vi "Lab Panel V5.11.vi"() -> ()   [LabVIEW 2013] (continued)
                      tunnel: w5311 -> [w5327 _]
                      tunnel: [w5326 FALSE] -> w5294
                      frame False {
                        n2899 = Equal?(x=w5328, y=w5327) -> (x = y?=w5326:bool)
                      }
                      frame True {
                      }
                    }
                    n2900 = Or(x=w5295, y=w5294) -> (x .or. y?=w5289:bool)
                    n2901 = Or(x=w5293, y=w5292) -> (x .or. y?=w5288:bool)
                    n2902 = Or(x=w5296, y=w5297) -> (x .or. y?=w5284:bool)
                    n2903 = Or(x=w5289, y=w5288) -> (x .or. y?=w5287:bool)
                    n2904 = Or(x=w5286, y=w5287) -> (x .or. y?=w5285:bool)
                    n2905 = Or(x=w5285, y=w5284) -> (x .or. y?=w5283:bool)
                  }
                  frame #3 {
                    n2906 = local read "on loops"() -> (w5366:dbl)
                    n2907 = local read "jig cycle"() -> (w5363:dbl)
                    n2908 = local read "Send Mail Now"() -> (w5357:bool)
                    n2909 = Add(x=w5366, y=3.0) -> (x+y=w5364:dbl)
                    n2910 = Equal?(x=w5363, y=w5364) -> (x = y?=w5358:bool)
                    n2911 = And(x=w5358, y=w5357) -> (x .and. y?=w5356:bool)
                    n2912 = And(x=w5362, y=w5358) -> (x .and. y?=w5361:bool)
                    n2913 = And(x=w5361, y=w5360) -> (x .and. y?=w5359:bool)
                    n2914 = Or(x=w5359, y=w5356) -> (x .or. y?=w5355:bool)
                    n2915 = case shown="True" w5355 {
                      tunnel: w5371 -> [_ w5377]
                      tunnel: w5370 -> [_ w5376]
                      tunnel: "Lab Panel Test Status" -> [_ w5375]
                      tunnel: w5368 -> [_ w5374]
                      tunnel: w5367 -> [_ w5373]
                      tunnel: w5354 -> [_ w5372]
                      frame False {
                      }
                      frame True {
                        n2916 = stacked-sequence {
                          tunnel: w5377 -> [w5385 _]
                          tunnel: w5376 -> [w5384 _]
                          tunnel: w5375 -> [w5383 _]
                          tunnel: w5374 -> [w5382 _]
                          tunnel: w5373 -> [w5381 _]
                          tunnel: w5372 -> [w5380 _]
                          frame #0 {
                            n2917 = call "sub vi - send mail v5.vi"("TO:"=w5385, "subject"=w5383, "from"=w5381, "out going server"=w5382, "message"=w5384) -> ("error out"=w5379:errorcluster)  [unwired: 10 in]
                            n2918 = Bundle(cluster=w5380, "mail error"=w5379) -> (w5378:T7)  [unwired: 6 in]
                            n2919 = local write "MAIL SETTINGS"(w5378) -> ()
                          }
                          frame #1 {
                            n2920 = local write "mail control"("") -> ()
                            n2921 = local write "Send Mail Now"(FALSE) -> ()
                          }
                        }
                      }
                    }
                  }
                }
              }
            }
          }
          frame #18 {
            # "save jig cycle values once all run switches are off"
            n2922 = stacked-sequence {
              tunnel: w5397 -> [_ w5426]
              tunnel: w5396 -> [_ w5425]
              tunnel: w5395 -> [_ w5424]
              tunnel: w5394 -> [_ w5423]
              tunnel: w5393 -> [_ w5422]
              tunnel: w5392 -> [_ w5421]
              tunnel: w5391 -> [_ w5420]
              tunnel: w5390 -> [_ w5419]
              tunnel: w5389 -> [_ w5418]
              tunnel: w5388 -> [_ w5417]
              frame #0 {
              }
              frame #1 {
                n2923 = Not(x=w5417) -> (.not. x?=w5400:bool)
                n2924 = Not(x=w5425) -> (.not. x?=w5415:bool)
                n2925 = Not(x=w5422) -> (.not. x?=w5410:bool)
                n2926 = Not(x=w5420) -> (.not. x?=w5406:bool)
                n2927 = Not(x=w5418) -> (.not. x?=w5402:bool)
                n2928 = Not(x=w5426) -> (.not. x?=w5416:bool)
                n2929 = Not(x=w5424) -> (.not. x?=w5414:bool)
                n2930 = Not(x=w5421) -> (.not. x?=w5408:bool)
                n2931 = Not(x=w5423) -> (.not. x?=w5412:bool)
                n2932 = Not(x=w5419) -> (.not. x?=w5404:bool)
                n2933 = local read "Save JC"() -> (w5428:bool)
                n2934 = And(x=w5416, y=w5415) -> (x .and. y?=w5413:bool)
                n2935 = And(x=w5413, y=w5414) -> (x .and. y?=w5411:bool)
                n2936 = And(x=w5411, y=w5412) -> (x .and. y?=w5409:bool)
                n2937 = And(x=w5409, y=w5410) -> (x .and. y?=w5407:bool)
                n2938 = And(x=w5407, y=w5408) -> (x .and. y?=w5405:bool)
                n2939 = And(x=w5405, y=w5406) -> (x .and. y?=w5403:bool)
                n2940 = And(x=w5403, y=w5404) -> (x .and. y?=w5401:bool)
                n2941 = And(x=w5401, y=w5402) -> (x .and. y?=w5399:bool)
                n2942 = And(x=w5399, y=w5400) -> (x .and. y?=w5398:bool)
                n2943 = And(x=w5398, y=w5428) -> (x .and. y?=w5427:bool)
                n2944 = case shown="True" w5427 {
                  tunnel: w5398 -> [w5429 _]
                  frame False {
                    n2945 = case shown="False" w5429 {
                      frame False {
                        n2946 = local write "Save JC"(TRUE) -> ()
                      }
                      frame True {
                      }
                    }
                  }
                  frame True {
                    n2947 = stacked-sequence {
                      frame #0 {
                        n2948 = String To Path(string="c:\\crabtree\\Jig Cycles\\") -> (path=w5441:path)
                        n2949 = Build Path(base path=w5441, name or relative path="jigcycles.bin") -> (appended path=w5439:path)
                        n2950 = Create Folder(path (use dialog)=w5441) -> (error out=w5443:errorcluster)  [unwired: 2 in, 2 out]
                        n2951 = local read "JIG RELAY CYCLES"() -> (w5433:T8)
                        n2952 = call <vilib>:"Clear Errors.vi"("error in (no error)"=w5443) -> ()  [unwired: 6 in, 1 out]
                        n2953 = local write "Save JC"(FALSE) -> ()
                        n2954 = Open/Create/Replace File(file path (use dialog)=w5439, operation (0:open)=T21."replace or create") -> (refnum out=w5437:refnum<file>, error out=w5438:errorcluster)  [unwired: 4 in, 1 out]
                        n2955 = Write to Binary File(file (use dialog)=w5437, data=w5433, error in=w5438) -> (refnum out=w5436:refnum<file>, error out=w5435:errorcluster)  [unwired: 3 in, 1 out]
                        n2956 = Close File(refnum=w5436, error in=w5435) -> (error out=w5434:errorcluster)  [unwired: 1 out]
                        n2957 = local write "data file error"(w5434) -> ()
                      }
                      frame #1 {
                        n2958 = local read "JIG RELAY CYCLES"() -> (w5466:T8)
                        n2959 = Unbundle By Name(w5466) -> ("LAB01-1"=w5461:dbl, "LAB01-2"=w5460:dbl, "LAB02-1"=w5458:dbl, "LAB02-2"=w5457:dbl, "LAB03-1"=w5455:dbl, "LAB03-2"=w5452:dbl, "LAB04-1"=w5451:dbl, "LAB04-2"=w5449:dbl, "LAB05-1"=w5447:dbl, "LAB05-2"=w5445:dbl)
                        n2960 = stacked-sequence {
                          tunnel: w5461 -> [w5469 _ _ _ _ _ _ _ _ _]
                          tunnel: 1000000 -> [w5472 w5482 w5492 w5502 w5512 w5522 w5532 w5542 w5552 w5562]
                          tunnel: [w5470 _ _ _ _ _ _ _ _ _] -> w5464
                          tunnel: "TEST STATION HAS REACHED 1 MILLION CYCLES, REPLACE  CONTROL RELAYS" -> [w5468 w5480 w5490 w5500 w5510 w5520 w5530 w5540 w5550 w5560]
                          tunnel: [_ w5479 _ _ _ _ _ _ _ _] -> w5462
                          tunnel: w5460 -> [_ w5478 _ _ _ _ _ _ _ _]
                          tunnel: [_ _ w5489 _ _ _ _ _ _ _] -> w5459
                          tunnel: w5458 -> [_ _ w5488 _ _ _ _ _ _ _]
                          tunnel: w5457 -> [_ _ _ w5499 _ _ _ _ _ _]
                          tunnel: [_ _ _ w5498 _ _ _ _ _ _] -> w5456
                          tunnel: w5455 -> [_ _ _ _ w5509 _ _ _ _ _]
                          tunnel: [_ _ _ _ w5508 _ _ _ _ _] -> w5454
                          tunnel: [_ _ _ _ _ w5519 _ _ _ _] -> w5453
                          tunnel: w5452 -> [_ _ _ _ _ w5518 _ _ _ _]
                          tunnel: w5451 -> [_ _ _ _ _ _ w5529 _ _ _]
                          tunnel: [_ _ _ _ _ _ w5528 _ _ _] -> w5450
                          tunnel: w5449 -> [_ _ _ _ _ _ _ w5539 _ _]
                          tunnel: [_ _ _ _ _ _ _ w5538 _ _] -> w5448
                          tunnel: w5447 -> [_ _ _ _ _ _ _ _ w5549 _]
                          tunnel: [_ _ _ _ _ _ _ _ w5548 _] -> w5446
                          tunnel: w5445 -> [_ _ _ _ _ _ _ _ _ w5559]
                          tunnel: [_ _ _ _ _ _ _ _ _ w5558] -> w5444
                          frame #0 {
                            n2961 = Greater?(x=w5469, y=w5472) -> (0:w5471:bool)
                            n2962 = case shown="True" w5471 {
                              tunnel: [w5473 0] -> w5470
                              tunnel: w5469 -> [w5473 _]
                              tunnel: w5468 -> [_ w5474]
                              frame False {
                              }
                              frame True {
                                n2963 = Concatenate Strings("LA01-1 ", w5474) -> (w5477:string)
                                n2964 = One Button Dialog(message=w5477) -> ()  [unwired: 1 in, 1 out]
                              }
                            }
                          }
                          frame #1 {
                            n2965 = Greater?(x=w5478, y=w5482) -> (0:w5481:bool)
                            n2966 = case shown="True" w5481 {
                              tunnel: [w5483 0] -> w5479
                              tunnel: w5478 -> [w5483 _]
                              tunnel: w5480 -> [_ w5484]
                              frame False {
                              }
                              frame True {
                                n2967 = Concatenate Strings("LA01-2 ", w5484) -> (w5487:string)
                                n2968 = One Button Dialog(message=w5487) -> ()  [unwired: 1 in, 1 out]
                              }
                            }
                          }
                          frame #2 {
                            n2969 = Greater?(x=w5488, y=w5492) -> (0:w5491:bool)
                            n2970 = case shown="True" w5491 {
                              tunnel: [w5493 0] -> w5489
                              tunnel: w5488 -> [w5493 _]
                              tunnel: w5490 -> [_ w5494]
                              frame False {
                              }
                              frame True {
                                n2971 = Concatenate Strings("LA02-1 ", w5494) -> (w5497:string)
                                n2972 = One Button Dialog(message=w5497) -> ()  [unwired: 1 in, 1 out]
                              }
                            }
                          }
                          frame #3 {
                            n2973 = Greater?(x=w5499, y=w5502) -> (0:w5501:bool)
                            n2974 = case shown="True" w5501 {
                              tunnel: [w5503 0] -> w5498
                              tunnel: w5499 -> [w5503 _]
                              tunnel: w5500 -> [_ w5504]
                              frame False {
                              }
                              frame True {
                                n2975 = Concatenate Strings("LA02-2 ", w5504) -> (w5507:string)
                                n2976 = One Button Dialog(message=w5507) -> ()  [unwired: 1 in, 1 out]
                              }
                            }
                          }
                          frame #4 {
                            n2977 = Greater?(x=w5509, y=w5512) -> (0:w5511:bool)
                            n2978 = case shown="True" w5511 {
                              tunnel: [w5513 0] -> w5508
                              tunnel: w5509 -> [w5513 _]
                              tunnel: w5510 -> [_ w5514]
                              frame False {
                              }
                              frame True {
                                n2979 = Concatenate Strings("LA03-1 ", w5514) -> (w5517:string)
                                n2980 = One Button Dialog(message=w5517) -> ()  [unwired: 1 in, 1 out]
                              }
                            }
                          }
                          frame #5 {
                            n2981 = Greater?(x=w5518, y=w5522) -> (0:w5521:bool)
                            n2982 = case shown="True" w5521 {
                              tunnel: [w5523 0] -> w5519
                              tunnel: w5518 -> [w5523 _]
                              tunnel: w5520 -> [_ w5524]
                              frame False {
                              }
                              frame True {
                                n2983 = Concatenate Strings("LA03-2 ", w5524) -> (w5527:string)
                                n2984 = One Button Dialog(message=w5527) -> ()  [unwired: 1 in, 1 out]
                              }
                            }
                          }
                          frame #6 {
                            n2985 = Greater?(x=w5529, y=w5532) -> (0:w5531:bool)
                            n2986 = case shown="True" w5531 {
                              tunnel: [w5533 0] -> w5528
                              tunnel: w5529 -> [w5533 _]
                              tunnel: w5530 -> [_ w5534]
                              frame False {
                              }
                              frame True {
                                n2987 = Concatenate Strings("LA04-1 ", w5534) -> (w5537:string)
                                n2988 = One Button Dialog(message=w5537) -> ()  [unwired: 1 in, 1 out]
                              }
                            }
                          }
                          frame #7 {
                            n2989 = Greater?(x=w5539, y=w5542) -> (0:w5541:bool)
                            n2990 = case shown="True" w5541 {
                              tunnel: [w5543 0] -> w5538
                              tunnel: w5539 -> [w5543 _]
                              tunnel: w5540 -> [_ w5544]
                              frame False {
                              }
                              frame True {
                                n2991 = Concatenate Strings("LA04-2 ", w5544) -> (w5547:string)
                                n2992 = One Button Dialog(message=w5547) -> ()  [unwired: 1 in, 1 out]
                              }
                            }
                          }
                          frame #8 {
                            n2993 = Greater?(x=w5549, y=w5552) -> (0:w5551:bool)
                            n2994 = case shown="True" w5551 {
                              tunnel: [w5553 0] -> w5548
                              tunnel: w5549 -> [w5553 _]
                              tunnel: w5550 -> [_ w5554]
                              frame False {
                              }
                              frame True {
                                n2995 = Concatenate Strings("LA05-1 ", w5554) -> (w5557:string)
                                n2996 = One Button Dialog(message=w5557) -> ()  [unwired: 1 in, 1 out]
                              }
                            }
                          }
                          frame #9 {
                            n2997 = Greater?(x=w5559, y=w5562) -> (0:w5561:bool)
                            n2998 = case shown="True" w5561 {
                              tunnel: [w5563 0] -> w5558
                              tunnel: w5559 -> [w5563 _]
                              tunnel: w5560 -> [_ w5564]
                              frame False {
                              }
                              frame True {
                                n2999 = Concatenate Strings("LA05-2 ", w5564) -> (w5567:string)
                                n3000 = One Button Dialog(message=w5567) -> ()  [unwired: 1 in, 1 out]
                              }
                            }
                          }
                        }
                        n3001 = Bundle By Name(cluster=w5466, "LAB01-1"=w5464, "LAB01-2"=w5462, "LAB02-1"=w5459, "LAB02-2"=w5456, "LAB03-1"=w5454, "LAB03-2"=w5453, "LAB04-1"=w5450, "LAB04-2"=w5448, "LAB05-1"=w5446, "LAB05-2"=w5444) -> (w5465:T8)
                        n3002 = local write "JIG RELAY CYCLES"(w5465) -> ()
                      }
                    }
                  }
                }
              }
            }
          }
          frame #19 {
            # "get temperature values"
            n3003 = local read "Panel #"() -> (w5568:dbl)
            n3004 = local read "Simulate"() -> (w5581:bool)
            n3005 = local read "Temp Test Cal"() -> (w5578:dbl)
            n3006 = stacked-sequence {
              seq-local: [w5584 _] -> [_ w5627]
              tunnel: w5581 -> [_ w5641]
              tunnel: T14 {"1  (A) cal"=1.0, "1 (V) cal"=1.0, "1 (PF) cal"=1.0, "1 (TL) cal"=1.0, "1 (TN) cal"=1.0, "2 (A) cal"=1.0, "2 (V) cal"=1.0, "2 (PF) cal"=1.0, "2 (TL) cal"=1.0, "2 (TN) cal"=1.0} ("CAL LAB01") -> [_ w5640]
              tunnel: w5579 -> [_ w5639]
              tunnel: w5578 -> [_ w5638]
              tunnel: w5577 -> [_ w5637]
              tunnel: w5576 -> [_ w5636]
              tunnel: w5575 -> [_ w5635]
              tunnel: w5574 -> [_ w5634]
              tunnel: w5573 -> [_ w5633]
              tunnel: w5572 -> [_ w5632]
              tunnel: w5571 -> [_ w5631]
              tunnel: w5570 -> [_ w5630]
              tunnel: w5569 -> [_ w5629]
              tunnel: w5568 -> [_ w5628]
              frame #0 {
                n3007 = local read "Select COM port"() -> (w5585:refnum<visa-resource-name>)
                "COM port" <- w5585
                n3008 = global write "Global 1.vi" "COM port"(w5585) -> ()
                n3009 = global write "Global 1.vi" "tmp dly lps"("Temp Delay Lps") -> ()
                n3010 = global write "Global 1.vi" "dly value"("Temp Value") -> ()
                n3011 = local read "jig cycle"() -> (w5587:dbl)
                n3012 = local read "on loops"() -> (w5589:dbl)
                n3013 = Add(x=w5589, y=3) -> (x+y=w5590:dbl)
                n3014 = local read "Panel #"() -> (w5586:dbl)
                n3015 = Equal?(x=w5587, y=w5590) -> (x = y?=w5584:bool)
                n3016 = case shown="True" w5584 {
                  tunnel: w5586 -> [_ w5595]
                  frame False {
                  }
                  frame True {
                    n3017 = local read "Simulate"() -> (w5592:bool)
                    n3018 = case shown="1" w5595 {
                      tunnel: 1.0 -> [_ w5602 w5605 w5612 w5617 w5623]
                      tunnel: w5592 -> [_ w5598 w5604 w5610 w5618 w5622]
                      tunnel: [FALSE w5597 w5603 w5609 w5615 w5621] -> w5591
                      frame 0, Default {
                      }
                      frame 1 {
                        w5600 = FALSE
                        n3019 = call "sub vi - GET ALL TEMP v7.vi"("LA01-EN"=TRUE, "simulate"=w5598, "LA02-EN"=w5600, "LA03-EN"=w5600, "LA04-EN"=w5600, "LA05-EN"=w5600, "Gen Cal Value"=w5602) -> ("LA01 TEMP"=w5599:T24, "error"=w5597:bool)  [unwired: 3 in, 4 out]
                        n3020 = local write "LAB01 TEMP"(w5599) -> ()
                      }
                      frame 2 {
                        w5606 = FALSE
                        n3021 = call "sub vi - GET ALL TEMP v7.vi"("LA01-EN"=w5606, "simulate"=w5604, "LA02-EN"=TRUE, "LA03-EN"=w5606, "LA04-EN"=w5606, "LA05-EN"=w5606, "Gen Cal Value"=w5605) -> ("LA02 TEMP"=w5608:T24, "error"=w5603:bool)  [unwired: 3 in, 4 out]
                        n3022 = local write "LAB02 TEMP"(w5608) -> ()
                      }
                      frame 3 {
                        w5613 = FALSE
                        n3023 = call "sub vi - GET ALL TEMP v7.vi"("LA01-EN"=w5613, "simulate"=w5610, "LA02-EN"=w5613, "LA03-EN"=TRUE, "LA04-EN"=w5613, "LA05-EN"=w5613, "Gen Cal Value"=w5612) -> ("LA03 TEMP"=w5611:T24, "error"=w5609:bool)  [unwired: 3 in, 4 out]
                        n3024 = local write "LAB03 TEMP"(w5611) -> ()
                      }
                      frame 4 {
                        w5619 = FALSE
                        n3025 = call "sub vi - GET ALL TEMP v7.vi"("LA01-EN"=w5619, "simulate"=w5618, "LA02-EN"=w5619, "LA03-EN"=w5619, "LA04-EN"=TRUE, "LA05-EN"=w5619, "Gen Cal Value"=w5617) -> ("LA04 TEMP"=w5616:T24, "error"=w5615:bool)  [unwired: 3 in, 4 out]
                        n3026 = local write "LAB04 TEMP"(w5616) -> ()
                      }
                      frame 5 {
                        w5625 = FALSE
                        n3027 = call "sub vi - GET ALL TEMP v7.vi"("LA01-EN"=w5625, "simulate"=w5622, "LA02-EN"=w5625, "LA03-EN"=w5625, "LA04-EN"=w5625, "LA05-EN"=TRUE, "Gen Cal Value"=w5623) -> ("error"=w5621:bool, "LA05 TEMP"=w5624:T24)  [unwired: 3 in, 4 out]
                        n3028 = local write "LAB05 TEMP"(w5624) -> ()
                      }
                    }
                    "Error Temp" <- w5591
                    n3029 = local write "TEMP"(TRUE) -> ()
                  }
                }
              }
              frame #1 {
                n3030 = case shown="True" w5627 {
                  tunnel: w5641 -> [_ w5655]
                  tunnel: w5640 -> [_ w5654]
                  tunnel: w5639 -> [_ w5653]
                  tunnel: w5638 -> [_ w5652]
                  tunnel: w5637 -> [_ w5651]
                  tunnel: w5636 -> [_ w5650]
                  tunnel: w5635 -> [_ w5649]
                  tunnel: w5634 -> [_ w5648]
                  tunnel: w5633 -> [_ w5647]
                  tunnel: w5632 -> [_ w5646]
                  tunnel: w5631 -> [_ w5645]
                  tunnel: w5630 -> [_ w5644]
                  tunnel: w5629 -> [_ w5643]
                  tunnel: w5628 -> [_ w5642]
                  frame False {
                  }
                  frame True {
                    n3031 = case shown="1" w5642 {
                      tunnel: w5655 -> [_ w5668 w5713 w5758 w5803 w5848]
                      tunnel: w5654 -> [_ w5667 w5712 w5757 w5802 w5847]
                      tunnel: w5653 -> [_ w5657 _ _ _ _]
                      tunnel: w5652 -> [_ w5662 w5711 w5756 w5801 w5846]
                      tunnel: w5651 -> [_ w5656 _ _ _ _]
                      tunnel: w5650 -> [_ _ w5702 _ _ _]
                      tunnel: w5649 -> [_ _ w5701 _ _ _]
                      tunnel: w5648 -> [_ _ _ w5747 _ _]
                      tunnel: w5647 -> [_ _ _ w5746 _ _]
                      tunnel: w5646 -> [_ _ _ _ w5792 _]
                      tunnel: w5645 -> [_ _ _ _ w5791 _]
                      tunnel: w5644 -> [_ _ _ _ _ w5837]
                      tunnel: w5643 -> [_ _ _ _ _ w5836]
                      frame ..0 {
                      }
                      frame 1 {
                        n3032 = case shown="False" w5668 {
                          tunnel: [w5699 w5700] -> w5684
                          tunnel: w5667 -> [_ w5700]
                          frame False {
                            n3033 = local read "CAL LAB01"() -> (w5699:T14)
                          }
                          frame True {
                          }
                        }
                        n3034 = local read "TEMP LA01"() -> (w5675:T9)
                        n3035 = local read "LAB01 TEMP"() -> (w5674:T12)
                        n3036 = call "sub vi - temperature delay v3.vi"("2-run"=w5656, "1-run"=w5657, "temp values IN"=w5675, "temp signals"=w5674) -> ("T2-N"=w5670:dbl, "T2-L"=w5671:dbl, "T1-N"=w5672:dbl, "T1-L"=w5673:dbl, "temp values OUT"=w5669:T43)  [unwired: 3 in]
                        n3037 = Unbundle By Name(w5684) -> ("1 (TL) cal"=w5679:dbl, "1 (TN) cal"=w5678:dbl, "2 (TL) cal"=w5677:dbl, "2 (TN) cal"=w5676:dbl)  [unwired: 6 out]
                        n3038 = local write "TEMP LA01"(w5669) -> ()
                        n3039 = Multiply(x=w5673, y=w5679) -> (x*y=w5666:dbl)
                        n3040 = Multiply(x=w5672, y=w5678) -> (x*y=w5664:dbl)
                        n3041 = Multiply(x=w5671, y=w5677) -> (x*y=w5661:dbl)
                        n3042 = Multiply(x=w5670, y=w5676) -> (x*y=w5660:dbl)
                        n3043 = case shown="True" w5657 {
                          tunnel: w5666 -> [w5693 w5698]
                          tunnel: w5662 -> [_ w5696]
                          tunnel: [w5693 w5697] -> w5665
                          tunnel: w5664 -> [w5692 w5695]
                          tunnel: [w5692 w5694] -> w5663
                          frame False {
                          }
                          frame True {
                            n3044 = Multiply(x=w5696, y=w5695) -> (x*y=w5694:dbl)
                            n3045 = Multiply(x=w5696, y=w5698) -> (x*y=w5697:dbl)
                          }
                        }
                        n3046 = case shown="True" w5656 {
                          tunnel: w5661 -> [w5686 w5691]
                          tunnel: w5662 -> [_ w5689]
                          tunnel: [w5686 w5690] -> w5659
                          tunnel: w5660 -> [w5685 w5688]
                          tunnel: [w5685 w5687] -> w5658
                          frame False {
                          }
                          frame True {
                            n3047 = Multiply(x=w5689, y=w5688) -> (x*y=w5687:dbl)
                            n3048 = Multiply(x=w5689, y=w5691) -> (x*y=w5690:dbl)
                          }
                        }
                        n3049 = local read "SIG LAB01-2"() -> (w5681:T2)
                        n3050 = local read "SIG LAB01-1"() -> (w5683:T2)
                        n3051 = Bundle By Name(cluster=w5683, "Tmp Live"=w5665, "Tmp Neut"=w5663) -> (w5682:T2)
                        n3052 = Bundle By Name(cluster=w5681, "Tmp Live"=w5659, "Tmp Neut"=w5658) -> (w5680:T2)
                        n3053 = local write "SIG LAB01-1"(w5682) -> ()
                        n3054 = local write "SIG LAB01-2"(w5680) -> ()
                      }
                      frame 2 {
                        n3055 = case shown="True" w5713 {
                          tunnel: [w5744 w5745] -> w5729
                          tunnel: w5712 -> [_ w5745]
                          frame False {
                            n3056 = local read "CAL LAB02"() -> (w5744:T15)
                          }
                          frame True {
                          }
                        }
                        n3057 = local read "LAB02 TEMP"() -> (w5720:T12)
                        n3058 = local read "TEMP LA02"() -> (w5719:T9)
                        n3059 = call "sub vi - temperature delay v3.vi"("2-run"=w5701, "1-run"=w5702, "temp values IN"=w5719, "temp signals"=w5720) -> ("T2-N"=w5714:dbl, "T2-L"=w5715:dbl, "T1-N"=w5716:dbl, "T1-L"=w5717:dbl, "temp values OUT"=w5718:T43)  [unwired: 3 in]
                        n3060 = Unbundle By Name(w5729) -> ("1 (TL) cal"=w5724:dbl, "1 (TN) cal"=w5723:dbl, "2 (TL) cal"=w5722:dbl, "2 (TN) cal"=w5721:dbl)  [unwired: 6 out]
                        n3061 = local write "TEMP LA02"(w5718) -> ()
                        n3062 = Multiply(x=w5717, y=w5724) -> (x*y=w5710:dbl)
                        n3063 = Multiply(x=w5716, y=w5723) -> (x*y=w5709:dbl)
                        n3064 = Multiply(x=w5715, y=w5722) -> (x*y=w5706:dbl)
                        n3065 = Multiply(x=w5714, y=w5721) -> (x*y=w5705:dbl)
                        n3066 = case shown="True" w5702 {
                          tunnel: w5710 -> [w5738 w5743]
                          tunnel: w5711 -> [_ w5741]
                          tunnel: [w5738 w5742] -> w5708
                          tunnel: w5709 -> [w5737 w5740]
                          tunnel: [w5737 w5739] -> w5707
                          frame False {
                          }
                          frame True {
                            n3067 = Multiply(x=w5741, y=w5740) -> (x*y=w5739:dbl)
                            n3068 = Multiply(x=w5741, y=w5743) -> (x*y=w5742:dbl)
                          }
                        }
                        n3069 = case shown="True" w5701 {
                          tunnel: w5706 -> [w5731 w5736]
                          tunnel: w5711 -> [_ w5734]
                          tunnel: [w5731 w5735] -> w5704
                          tunnel: w5705 -> [w5730 w5733]
                          tunnel: [w5730 w5732] -> w5703
                          frame False {
                          }
                          frame True {
                            n3070 = Multiply(x=w5734, y=w5733) -> (x*y=w5732:dbl)
                            n3071 = Multiply(x=w5734, y=w5736) -> (x*y=w5735:dbl)
                          }
                        }
                        n3072 = local read "SIG LAB02-2"() -> (w5726:T2)
                        n3073 = local read "SIG LAB02-1"() -> (w5728:T2)
                        n3074 = Bundle By Name(cluster=w5728, "Tmp Live"=w5708, "Tmp Neut"=w5707) -> (w5727:T2)
                        n3075 = Bundle By Name(cluster=w5726, "Tmp Live"=w5704, "Tmp Neut"=w5703) -> (w5725:T2)
                        n3076 = local write "SIG LAB02-1"(w5727) -> ()
                        n3077 = local write "SIG LAB02-2"(w5725) -> ()
                      }
                      frame 3 {
                        n3078 = case shown="False" w5758 {
                          tunnel: [w5789 w5790] -> w5774
                          tunnel: w5757 -> [_ w5790]
                          frame False {
                            n3079 = local read "CAL LAB03"() -> (w5789:T14)
                          }
                          frame True {
                          }
                        }
                        n3080 = local read "TEMP LA03"() -> (w5764:T9)
                        n3081 = local read "LAB03 TEMP"() -> (w5765:T12)
                        n3082 = call "sub vi - temperature delay v3.vi"("2-run"=w5746, "1-run"=w5747, "temp values IN"=w5764, "temp signals"=w5765) -> ("T2-N"=w5759:dbl, "T2-L"=w5760:dbl, "T1-N"=w5761:dbl, "T1-L"=w5762:dbl, "temp values OUT"=w5763:T43)  [unwired: 3 in]
                        n3083 = Unbundle By Name(w5774) -> ("1 (TL) cal"=w5769:dbl, "1 (TN) cal"=w5768:dbl, "2 (TL) cal"=w5767:dbl, "2 (TN) cal"=w5766:dbl)  [unwired: 6 out]
                        n3084 = local write "TEMP LA03"(w5763) -> ()
                        n3085 = Multiply(x=w5762, y=w5769) -> (x*y=w5755:dbl)
                        n3086 = Multiply(x=w5761, y=w5768) -> (x*y=w5754:dbl)
                        n3087 = Multiply(x=w5760, y=w5767) -> (x*y=w5751:dbl)
                        n3088 = Multiply(x=w5759, y=w5766) -> (x*y=w5750:dbl)
                        n3089 = case shown="True" w5746 {
                          tunnel: w5751 -> [w5776 w5781]
                          tunnel: w5756 -> [_ w5779]
                          tunnel: [w5776 w5780] -> w5749
                          tunnel: w5750 -> [w5775 w5778]
                          tunnel: [w5775 w5777] -> w5748
                          frame False {
                          }
                          frame True {
                            n3090 = Multiply(x=w5779, y=w5778) -> (x*y=w5777:dbl)
                            n3091 = Multiply(x=w5779, y=w5781) -> (x*y=w5780:dbl)
                          }
                        }
                        n3092 = case shown="True" w5747 {
                          tunnel: w5755 -> [w5783 w5788]
                          tunnel: w5756 -> [_ w5786]
                          tunnel: [w5783 w5787] -> w5753
                          tunnel: w5754 -> [w5782 w5785]
                          tunnel: [w5782 w5784] -> w5752
                          frame False {
                          }
                          frame True {
                            n3093 = Multiply(x=w5786, y=w5785) -> (x*y=w5784:dbl)
                            n3094 = Multiply(x=w5786, y=w5788) -> (x*y=w5787:dbl)
                          }
                        }
                        n3095 = local read "SIG LAB03-2"() -> (w5771:T2)
                        n3096 = local read "SIG LAB03-1"() -> (w5773:T2)
                        n3097 = Bundle By Name(cluster=w5773, "Tmp Live"=w5753, "Tmp Neut"=w5752) -> (w5772:T2)
                        n3098 = Bundle By Name(cluster=w5771, "Tmp Live"=w5749, "Tmp Neut"=w5748) -> (w5770:T2)
                        n3099 = local write "SIG LAB03-1"(w5772) -> ()
                        n3100 = local write "SIG LAB03-2"(w5770) -> ()
                      }
                      frame 4 {
                        n3101 = case shown="False" w5803 {
                          tunnel: [w5834 w5835] -> w5819
                          tunnel: w5802 -> [_ w5835]
                          frame False {
                            n3102 = local read "CAL LAB04"() -> (w5834:T14)
                          }
                          frame True {
                          }
                        }
                        n3103 = local read "LAB04 TEMP"() -> (w5809:T12)
                        n3104 = local read "TEMP LA04"() -> (w5810:T9)
                        n3105 = call "sub vi - temperature delay v3.vi"("2-run"=w5791, "1-run"=w5792, "temp values IN"=w5810, "temp signals"=w5809) -> ("T2-N"=w5804:dbl, "T2-L"=w5805:dbl, "T1-N"=w5806:dbl, "T1-L"=w5807:dbl, "temp values OUT"=w5808:T43)  [unwired: 3 in]
                        n3106 = Unbundle By Name(w5819) -> ("1 (TL) cal"=w5814:dbl, "1 (TN) cal"=w5813:dbl, "2 (TL) cal"=w5812:dbl, "2 (TN) cal"=w5811:dbl)  [unwired: 6 out]
                        n3107 = local write "TEMP LA04"(w5808) -> ()
                        n3108 = Multiply(x=w5807, y=w5814) -> (x*y=w5800:dbl)
                        n3109 = Multiply(x=w5806, y=w5813) -> (x*y=w5799:dbl)
                        n3110 = Multiply(x=w5805, y=w5812) -> (x*y=w5796:dbl)
                        n3111 = Multiply(x=w5804, y=w5811) -> (x*y=w5795:dbl)
                        n3112 = case shown="True" w5791 {
                          tunnel: w5796 -> [w5821 w5826]
                          tunnel: w5801 -> [_ w5824]
                          tunnel: [w5821 w5825] -> w5794
                          tunnel: w5795 -> [w5820 w5823]
                          tunnel: [w5820 w5822] -> w5793
                          frame False {
                          }
                          frame True {
                            n3113 = Multiply(x=w5824, y=w5823) -> (x*y=w5822:dbl)
                            n3114 = Multiply(x=w5824, y=w5826) -> (x*y=w5825:dbl)
                          }
                        }
                        n3115 = case shown="True" w5792 {
                          tunnel: w5800 -> [w5828 w5833]
                          tunnel: w5801 -> [_ w5831]
                          tunnel: [w5828 w5832] -> w5798
                          tunnel: w5799 -> [w5827 w5830]
                          tunnel: [w5827 w5829] -> w5797
                          frame False {
                          }
                          frame True {
                            n3116 = Multiply(x=w5831, y=w5830) -> (x*y=w5829:dbl)
                            n3117 = Multiply(x=w5831, y=w5833) -> (x*y=w5832:dbl)
                          }
                        }
                        n3118 = local read "SIG LAB04-2"() -> (w5816:T2)
                        n3119 = local read "SIG LAB04-1"() -> (w5818:T2)
                        n3120 = Bundle By Name(cluster=w5818, "Tmp Live"=w5798, "Tmp Neut"=w5797) -> (w5817:T2)
                        n3121 = Bundle By Name(cluster=w5816, "Tmp Live"=w5794, "Tmp Neut"=w5793) -> (w5815:T2)
                        n3122 = local write "SIG LAB04-1"(w5817) -> ()
                        n3123 = local write "SIG LAB04-2"(w5815) -> ()
                      }
                      frame 5.. {
                        n3124 = case shown="False" w5848 {
                          tunnel: [w5879 w5880] -> w5864
                          tunnel: w5847 -> [_ w5880]
                          frame False {
                            n3125 = local read "CAL LAB05"() -> (w5879:T14)
                          }
                          frame True {
                          }
                        }
                        n3126 = local read "LAB05 TEMP"() -> (w5854:T12)
                        n3127 = local read "TEMP LA05"() -> (w5855:T9)
                        n3128 = call "sub vi - temperature delay v3.vi"("2-run"=w5836, "1-run"=w5837, "temp values IN"=w5855, "temp signals"=w5854) -> ("T2-N"=w5850:dbl, "T2-L"=w5851:dbl, "T1-N"=w5852:dbl, "T1-L"=w5853:dbl, "temp values OUT"=w5849:T43)  [unwired: 3 in]
                        n3129 = local write "TEMP LA05"(w5849) -> ()
                        n3130 = Unbundle By Name(w5864) -> ("1 (TL) cal"=w5856:dbl, "1 (TN) cal"=w5859:dbl, "2 (TL) cal"=w5858:dbl, "2 (TN) cal"=w5857:dbl)  [unwired: 6 out]
                        n3131 = Multiply(x=w5853, y=w5856) -> (x*y=w5845:dbl)
                        n3132 = Multiply(x=w5852, y=w5859) -> (x*y=w5844:dbl)
                        n3133 = Multiply(x=w5851, y=w5858) -> (x*y=w5841:dbl)
                        n3134 = Multiply(x=w5850, y=w5857) -> (x*y=w5840:dbl)
                        n3135 = case shown="True" w5836 {
                          tunnel: w5841 -> [w5866 w5871]
                          tunnel: w5846 -> [_ w5869]
                          tunnel: [w5866 w5870] -> w5839
                          tunnel: w5840 -> [w5865 w5868]
                          tunnel: [w5865 w5867] -> w5838
                          frame False {
                          }
                          frame True {
                            n3136 = Multiply(x=w5869, y=w5868) -> (x*y=w5867:dbl)
                            n3137 = Multiply(x=w5869, y=w5871) -> (x*y=w5870:dbl)
                          }
                        }
                        n3138 = case shown="True" w5837 {
                          tunnel: w5845 -> [w5873 w5878]
                          tunnel: w5846 -> [_ w5876]
                          tunnel: [w5873 w5877] -> w5843
                          tunnel: w5844 -> [w5872 w5875]
                          tunnel: [w5872 w5874] -> w5842
                          frame False {
                          }
                          frame True {
                            n3139 = Multiply(x=w5876, y=w5875) -> (x*y=w5874:dbl)
                            n3140 = Multiply(x=w5876, y=w5878) -> (x*y=w5877:dbl)
                          }
                        }
                        n3141 = local read "SIG LAB05-1"() -> (w5863:T2)
                        n3142 = Bundle By Name(cluster=w5863, "Tmp Live"=w5843, "Tmp Neut"=w5842) -> (w5862:T2)
                        n3143 = local read "SIG LAB05-2"() -> (w5861:T2)
                        n3144 = Bundle By Name(cluster=w5861, "Tmp Live"=w5839, "Tmp Neut"=w5838) -> (w5860:T2)
                        n3145 = local write "SIG LAB05-1"(w5862) -> ()
                        n3146 = local write "SIG LAB05-2"(w5860) -> ()
                      }
                    }
                  }
                }
              }
            }
          }
          frame #20 {
            # "write data to display panel"
            n3147 = global write "Global display 1.vi" "TEST 5-2"(w5915) -> ()
            n3148 = global write "Global display 1.vi" "TEST 4-2"(w5917) -> ()
            n3149 = global write "Global display 1.vi" "TEST 1-2"(w5923) -> ()
            n3150 = global write "Global display 1.vi" "TEST 3-1"(w5920) -> ()
            n3151 = global write "Global display 1.vi" "TEST 5-1"(w5916) -> ()
            n3152 = global write "Global display 1.vi" "TEST 1-1"(w5924) -> ()
            n3153 = global write "Global display 1.vi" "TEST 3-2"(w5919) -> ()
            n3154 = global write "Global display 1.vi" "TEST 4-1"(w5918) -> ()
            n3155 = global write "Global display 1.vi" "TEST 2-2"(w5921) -> ()
            n3156 = global write "Global display 1.vi" "TEST 2-1"(w5922) -> ()
            n3157 = global read "Global display 3.vi" "log 1-1"() -> (→"LOG LAB01-1":string)
            n3158 = global read "Global display 3.vi" "log 3-1"() -> (→"LOG LAB03-1":string)
            n3159 = global read "Global display 3.vi" "log 1-2"() -> (→"LOG LAB01-2":string)
            n3160 = property on="Tab Control 2" class="TabCtl (strict)"() -> ("Pages"=w5914:refnum<vi>[])  [unwired: 2 in, 2 out]
            n3161 = global read "Global display 3.vi" "log 2-1"() -> (→"LOG LAB02-1":string)
            n3162 = global read "Global display 3.vi" "log 2-2"() -> (→"LOG LAB02-2":string)
            n3163 = global read "Global display 3.vi" "log 4-2"() -> (→"LOG LAB04-2":string)
            n3164 = global read "Global display 3.vi" "log 5-2"() -> (→"LOG LAB05-2":string)
            n3165 = global read "Global display 3.vi" "log 5-1"() -> (→"LOG LAB05-1":string)
            n3166 = global read "Global display 3.vi" "log 4-1"() -> (→"LOG LAB04-1":string)
            n3167 = global read "Global display 3.vi" "log 3-2"() -> (→"LOG LAB03-2":string)
            n3168 = Index Array(array=w5914, index=8) -> (element=w5912:refnum<vi>)
            n3169 = property class="Page"(reference=w5912) -> ("PageVis"=w5911:bool)  [unwired: 1 in, 2 out]
            n3170 = global write "Global display 3.vi" "admin"(w5911) -> ()
            n3171 = local read "O/I  LAB05-2"() -> (w5965:bool)
            n3172 = local read "O/I  LAB05-1"() -> (w5966:bool)
            n3173 = local read "O/I  LAB03-2"() -> (w5969:bool)
            n3174 = local read "O/I  LAB04-2"() -> (w5967:bool)
            n3175 = local read "O/I  LAB04-1"() -> (w5968:bool)
            n3176 = local read "O/I  LAB03-1"() -> (w5970:bool)
            n3177 = local read "O/I  LAB01-2"() -> (w5973:bool)
            n3178 = local read "O/I  LAB01-1"() -> (w5974:bool)
            n3179 = local read "O/I  LAB02-1"() -> (w5972:bool)
            n3180 = local read "O/I  LAB02-2"() -> (w5971:bool)
            n3181 = global write "Global display 1.vi" "5-2 O/F"(w5965) -> ()
            n3182 = global write "Global display 1.vi" "5-1 O/F"(w5966) -> ()
            n3183 = global write "Global display 1.vi" "4-1 O/F"(w5968) -> ()
            n3184 = global write "Global display 1.vi" "4-2 O/F"(w5967) -> ()
            n3185 = global write "Global display 1.vi" "3-2 O/F"(w5969) -> ()
            n3186 = global write "Global display 1.vi" "3-1 O/F"(w5970) -> ()
            n3187 = global write "Global display 1.vi" "2-2 O/F"(w5971) -> ()
            n3188 = global write "Global display 1.vi" "2-1 O/F"(w5972) -> ()
            n3189 = global write "Global display 1.vi" "1-2 O/F"(w5973) -> ()
            n3190 = global write "Global display 1.vi" "1-1 O/F"(w5974) -> ()
            n3191 = local read "TEMP START LAB02-2"() -> (w5897:cluster{"TL":dbl, "TN":dbl})
            n3192 = local read "run lab05-2"() -> (w5955:bool)
            n3193 = local read "TEMP START LAB01-2"() -> (w5899:cluster{"TL":dbl, "TN":dbl})
            n3194 = local read "TEMP START LAB02-1"() -> (w5898:cluster{"TL":dbl, "TN":dbl})
            n3195 = local read "TEMP START LAB04-1"() -> (w5894:cluster{"TL":dbl, "TN":dbl})
            n3196 = local read "TEMP START LAB04-2"() -> (w5893:cluster{"TL":dbl, "TN":dbl})
            n3197 = local read "run lab04-1"() -> (w5958:bool)
            n3198 = local read "run lab04-2"() -> (w5957:bool)
            n3199 = local read "run lab05-1"() -> (w5956:bool)
            n3200 = local read "TEMP START LAB01-1"() -> (w5900:cluster{"TL":dbl, "TN":dbl})
            n3201 = local read "TEMP START LAB05-2"() -> (w5891:cluster{"TL":dbl, "TN":dbl})
            n3202 = local read "TEMP START LAB05-1"() -> (w5892:cluster{"TL":dbl, "TN":dbl})
            n3203 = local read "run lab03-2"() -> (w5959:bool)
            n3204 = local read "TEMP START LAB03-2"() -> (w5895:cluster{"TL":dbl, "TN":dbl})
            n3205 = local read "TEMP START LAB03-1"() -> (w5896:cluster{"TL":dbl, "TN":dbl})
            n3206 = local read "run lab02-1"() -> (w5962:bool)
            n3207 = local read "run lab03-1"() -> (w5960:bool)
            n3208 = local read "run lab01-2"() -> (w5963:bool)
            n3209 = local read "run lab02-2"() -> (w5961:bool)
            n3210 = local read "run lab01-1"() -> (w5964:bool)
            n3211 = global write "Global display 1.vi" "5-2 R/S"(w5955) -> ()
            n3212 = global write "Global display 1.vi" "5-1 R/S"(w5956) -> ()
            n3213 = global write "Global display 1.vi" "4-2 R/S"(w5957) -> ()
            n3214 = global write "Global display 1.vi" "4-1 R/S"(w5958) -> ()
            n3215 = global write "Global display 1.vi" "3-2 R/S"(w5959) -> ()
            n3216 = global write "Global display 1.vi" "1-2 R/S"(w5963) -> ()
            n3217 = global write "Global display 1.vi" "2-1 R/S"(w5962) -> ()
            n3218 = global write "Global display 1.vi" "3-1 R/S"(w5960) -> ()
            n3219 = global write "Global display 1.vi" "2-2 R/S"(w5961) -> ()
            n3220 = global write "Global display 1.vi" "1-1 R/S"(w5964) -> ()
            n3221 = global write "Global display 3.vi" "TEMP ST 05-2"(w5891) -> ()
            n3222 = global write "Global display 3.vi" "TEMP ST 05-1"(w5892) -> ()
            n3223 = global write "Global display 3.vi" "TEMP ST 03-2"(w5895) -> ()
            n3224 = global write "Global display 3.vi" "TEMP ST 04-2"(w5893) -> ()
            n3225 = global write "Global display 3.vi" "TEMP ST 01-1"(w5900) -> ()
            n3226 = global write "Global display 3.vi" "TEMP ST 01-2"(w5899) -> ()
            n3227 = global write "Global display 3.vi" "TEMP ST 04-1"(w5894) -> ()
            n3228 = global write "Global display 3.vi" "TEMP ST 02-1"(w5898) -> ()
            n3229 = global write "Global display 3.vi" "TEMP ST 02-2"(w5897) -> ()
            n3230 = global write "Global display 3.vi" "TEMP ST 03-1"(w5896) -> ()
            n3231 = local read "DISP LAB04-2"() -> (w5947:T4)
            n3232 = local read "DISP LAB05-1"() -> (w5946:T4)
            n3233 = local read "DISP LAB04-1"() -> (w5948:T4)
            n3234 = local read "DISP LAB05-2"() -> (w5945:T4)
            n3235 = local read "DISP LAB03-1"() -> (w5950:T4)
            n3236 = local read "DISP LAB03-2"() -> (w5949:T4)
            n3237 = local read "DISP LAB01-2"() -> (w5953:T4)
            n3238 = local read "DISP LAB02-1"() -> (w5952:T4)
            n3239 = local read "DISP LAB02-2"() -> (w5951:T4)
            n3240 = local read "DISP LAB01-1"() -> (w5954:T4)
            n3241 = local read "TEMP RISE LAB05-1"() -> (w5882:cluster{"TL":dbl, "TN":dbl})
            n3242 = local read "TEMP RISE LAB05-2"() -> (w5881:cluster{"TL":dbl, "TN":dbl})
            n3243 = local read "TEMP RISE LAB04-2"() -> (w5883:cluster{"TL":dbl, "TN":dbl})
            n3244 = local read "TEMP RISE LAB04-1"() -> (w5884:cluster{"TL":dbl, "TN":dbl})
            n3245 = local read "TEMP RISE LAB03-2"() -> (w5885:cluster{"TL":dbl, "TN":dbl})
            n3246 = local read "TEMP RISE LAB03-1"() -> (w5886:cluster{"TL":dbl, "TN":dbl})
            n3247 = local read "TEMP RISE LAB01-2"() -> (w5889:cluster{"TL":dbl, "TN":dbl})
            n3248 = local read "TEMP RISE LAB02-2"() -> (w5887:cluster{"TL":dbl, "TN":dbl})
            n3249 = local read "TEMP RISE LAB01-1"() -> (w5890:cluster{"TL":dbl, "TN":dbl})
            n3250 = local read "TEMP RISE LAB02-1"() -> (w5888:cluster{"TL":dbl, "TN":dbl})
            n3251 = global write "Global display 2.vi" "DISP LAB05-1"(w5946) -> ()
            n3252 = global write "Global display 2.vi" "DISP LAB05-2"(w5945) -> ()
            n3253 = global write "Global display 2.vi" "DISP LAB04-2"(w5947) -> ()
            n3254 = global write "Global display 2.vi" "DISP LAB02-1"(w5952) -> ()
            n3255 = global write "Global display 2.vi" "DISP LAB02-2"(w5951) -> ()
            n3256 = global write "Global display 2.vi" "DISP LAB04-1"(w5948) -> ()
            n3257 = global write "Global display 2.vi" "DISP LAB01-2"(w5953) -> ()
            n3258 = global write "Global display 2.vi" "DISP LAB01-1"(w5954) -> ()
            n3259 = global write "Global display 2.vi" "DISP LAB03-1"(w5950) -> ()
            n3260 = global write "Global display 2.vi" "DISP LAB03-2"(w5949) -> ()
            n3261 = global write "Global display 3.vi" "TEMP RS 05-2"(w5881) -> ()
            n3262 = global write "Global display 3.vi" "TEMP RS 05-1"(w5882) -> ()
            n3263 = global write "Global display 3.vi" "TEMP RS 03-2"(w5885) -> ()
            n3264 = global write "Global display 3.vi" "TEMP RS 02-1"(w5888) -> ()
            n3265 = global write "Global display 3.vi" "TEMP RS 02-2"(w5887) -> ()
            n3266 = global write "Global display 3.vi" "TEMP RS 04-2"(w5883) -> ()
            n3267 = global write "Global display 3.vi" "TEMP RS 01-2"(w5889) -> ()
            n3268 = global write "Global display 3.vi" "TEMP RS 03-1"(w5886) -> ()
            n3269 = global write "Global display 3.vi" "TEMP RS 04-1"(w5884) -> ()
            n3270 = global write "Global display 3.vi" "TEMP RS 01-1"(w5890) -> ()
